vi "Do.vi"(8 "error in":errorcluster, 10 "Actor in":refnum<class "Actor.lvclass">, 11 "EDS File Loaded Msg":refnum<class "EDS File Loaded Msg.lvclass">) -> (0 "error out":errorcluster, 2 "Actor out":refnum<class "Actor.lvclass">)   [LabVIEW 2020, in "Home.lvlib" / "EDS File Loaded Msg.lvclass"]
doc: "This VI delivers the message to the actor by calling the appropriate method(s) on the actor."
uses:
  EDS File Loaded Msg.lvclass
  <vilib>/ActorFramework/Actor/Actor.lvclass
  EDS File Loaded Msg.lvclass/EDS File Loaded Msg.ctl
  Home/Home.lvclass
  C:/Program Files/National Instruments/LabVIEW 2026/vi.lib/ActorFramework/Actor/Actor.lvclass
  9ef47adc-f318-494c-9b8b-6df3216d6863.vi
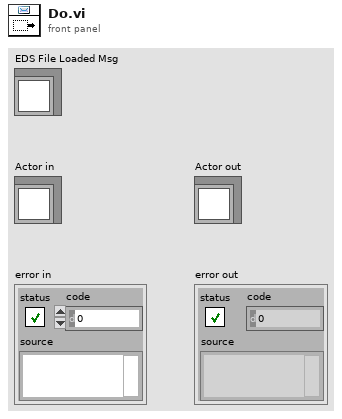
[diagram p1: front panel]
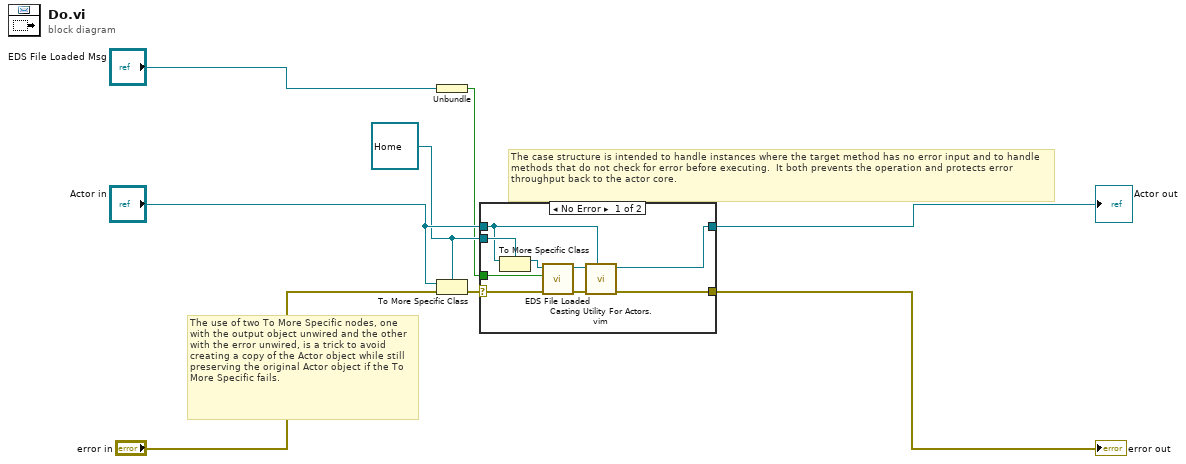
[diagram p0: block diagram]
diagram:
  w2 = refnum<class "Home.lvclass"> refnum ("Actor in")
  # "The use of two To More Specific nodes, one with the output object unwired and the other with the error unwired, is a trick to avoid creating a copy of the Actor object while still preserving the original Actor object if the To More Specific fails."
  # "The case structure is intended to handle instances where the target method has no error input and to handle methods that do not check for error before executing.  It both prevents the operation and protects error throughput back to the actor core."
  n1 = Unbundle("EDS File Loaded Msg") -> (w1:bool)
  n2 = To More Specific Class(target class=w2, reference="Actor in", error in="error in") -> (error out=w7:errorcluster)  [unwired: 1 out]
  n3 = case shown="No Error" w7 {
    selector: w7 -> [w17 w19]
    tunnel: [w16 w19] -> w6
    tunnel: [w10 w18] -> w4
    tunnel: "Actor in" -> [w12 w18]
    tunnel: w2 -> [w13 _]
    tunnel: w1 -> [w9 _]
    frame No Error {
      n4 = To More Specific Class(target class=w13, reference=w12) -> (specific class reference=w14:refnum<class "Home.lvclass">)  [unwired: 1 in, 1 out]
      n5 = call-dynamic "EDS File Loaded.vi"("error in"=w17, "Valid?"=w9, "Home in"=w14) -> ("error out"=w15:errorcluster, "Home out"=w11:refnum<class "Home.lvclass">)  [unwired: 7 in]
      n6 = call "Casting Utility For Actors.vim"("type"=w12, "error in (no error)"=w15, "Actor in"=w11) -> ("error out"=w16:errorcluster, "Actor out"=w10:refnum<class "Actor.lvclass">)  [unwired: 7 in]
    }
    frame Error {
      # "If type check fails, pass the original object out again."
    }
  }
  "error out" <- w6
  "Actor out" <- w4
